vi "Save Report.vi"(8 "error in (no error)":errorcluster, 10 "Report File Path":path) -> (0 "error out":errorcluster)   [LabVIEW 2020, in "Astemes_CSVReportPlugin.lvlib" / "Report Generator.lvlib"]
uses:
  Report Generator.lvlib
  Private/Reference.vi
  Test Result Handler/TestStand Result Handler.lvclass
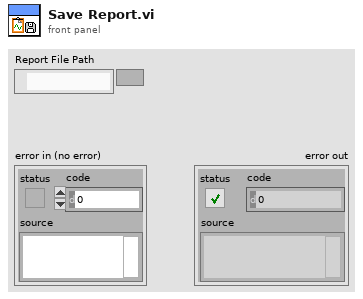
[diagram p1: front panel]
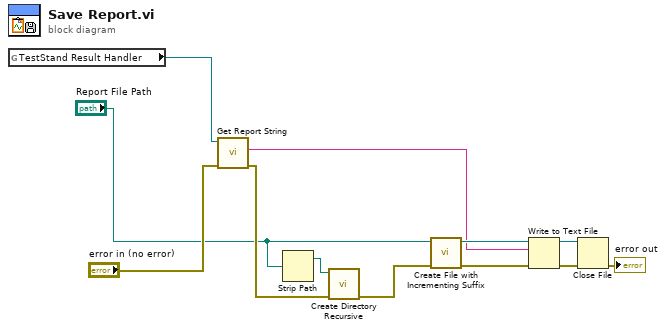
[diagram p0: block diagram]
diagram:
  n1 = global read "Reference.vi" "TestStand Result Handler"() -> (w12:refnum<class "TestStand Result Handler.lvclass">)
  n2 = call "Get Report String.vi"("error in (no error)"="error in (no error)", "TestStand Result Handler In"=w12) -> ("error out"=w11:errorcluster, "Report Text"=w4:string)  [unwired: 8 in]
  n3 = Strip Path(path="Report File Path") -> (stripped path=w1:path)  [unwired: 1 out]
  n4 = call <vilib>:"Create Directory Recursive.vi"("error in (no error)"=w11, "directory"=w1) -> ("error out"=w3:errorcluster)  [unwired: 3 in, 2 out]
  n5 = call <vilib>:"Create File with Incrementing Suffix.vi"("error in (no error)"=w3, "file path"="Report File Path") -> ("error out"=w9:errorcluster, "refnum out"=w6:refnum<file>)  [unwired: 7 in, 1 out]
  n6 = Write to Text File(file (use dialog)=w6, text=w4, error in=w9) -> (refnum out=w5:refnum<file>, error out=w8:errorcluster)  [unwired: 1 in, 1 out]
  n7 = Close File(refnum=w5, error in=w8) -> (error out=→"error out":errorcluster)  [unwired: 1 out]
